vi "Pockels_FPGA.vi"(6 "Ethernet Port Opened ?":bool, 8 "error in (no error)":errorcluster, 9 "Laser(V)":dbl format="%#_13g", 10 "Pockels Mode_FPGA":T1(ring)=enum."Modulate", 11 "Imaging Protocol":T2=enum."Live Imaging") -> (0 "error out":errorcluster, 3 "Pockels Packet":string)   [LabVIEW 2020]
uses:
  Typedefs/Imaging Protocols enum.ctl
  Global Variables/General Globals.vi
panel:
  out "number":u32
  out "bin_in":bool[](array[boolean])
  out "bin_out_invert_14":bool[](array[boolean])
  out "Hex string 2":string
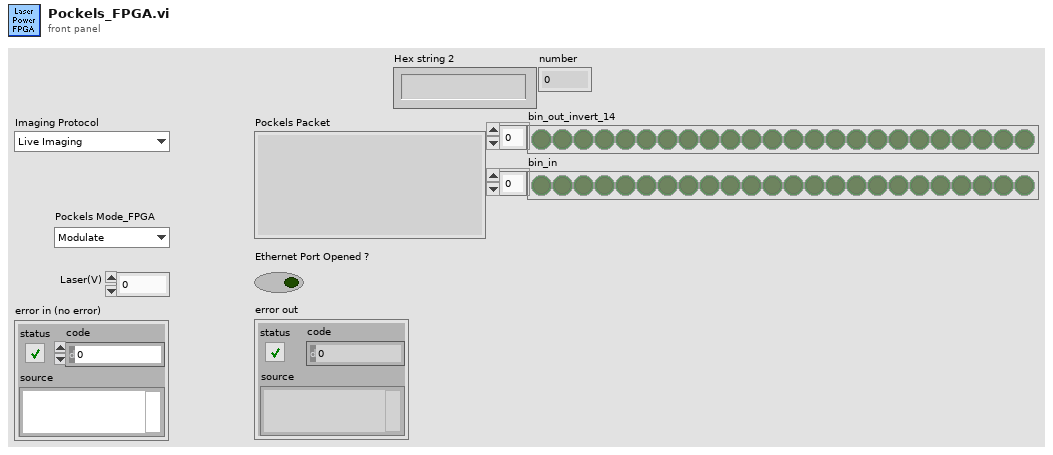
[diagram p1: front panel]
types:
  T1 = enum8{"Clear the register", "Always ON", "Modulate"}
  T2 = typedef "Imaging Protocols enum.ctl" = enum16{"AOL Z-Stack", "Motor Z Stack", "Functional Acquisition", "Single Plane Acquisition", "Volume Acquisition", "Live Imaging", "Live Plane Imaging", "Live Volume Imaging"}
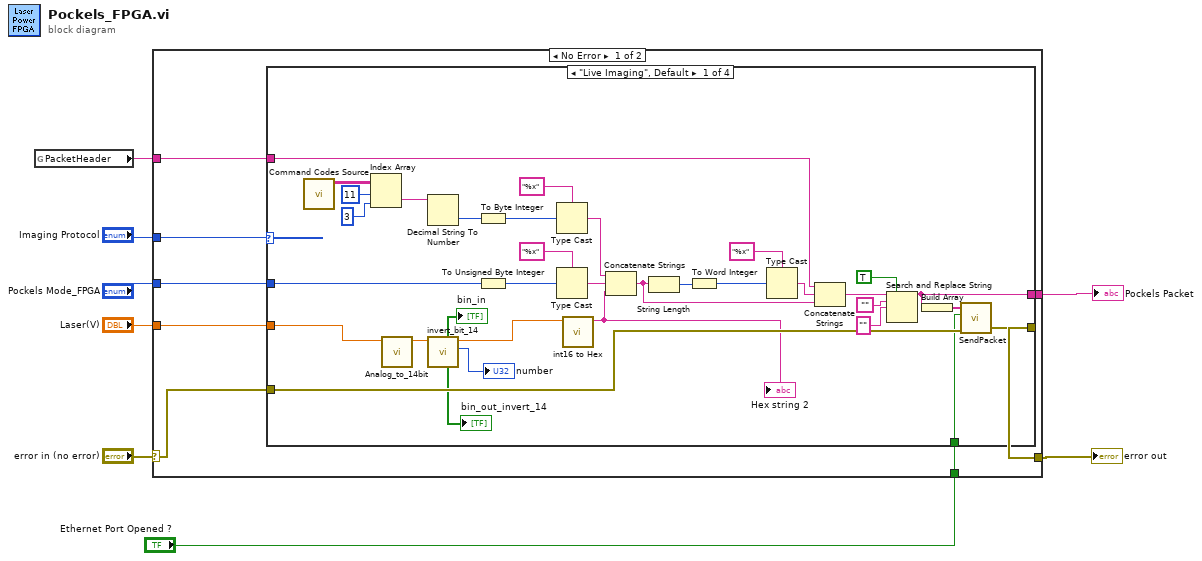
[diagram p0: block diagram]
diagram:
  n1 = global read "General Globals.vi" "PacketHeader"() -> (w3:string)
  n2 = case shown="No Error" "error in (no error)" {
    selector: "error in (no error)" -> [w10 w54]
    tunnel: "Imaging Protocol" -> [w16 _]
    tunnel: [w11 w54] -> w6
    tunnel: "Laser(V)" -> [w15 _]
    tunnel: "Pockels Mode_FPGA" -> [w14 _]
    tunnel: w3 -> [w13 _]
    tunnel: [w12 _] -> w2
    tunnel: "Ethernet Port Opened ?" -> [w9 _]
    frame No Error {
      n3 = case shown="\"Live Imaging\", Default" w16 {
        tunnel: w15 -> [w23 _ _ _]
        tunnel: w14 -> [w30 _ _ _]
        tunnel: w13 -> [w29 _ _ _]
        tunnel: [w27 _ _ _] -> w12
        tunnel: [w26 w51 w52 w53] -> w11
        tunnel: w10 -> [w25 w51 w52 w53]
        tunnel: w9 -> [w17 _ _ _]
        frame "Live Imaging", Default {
          n4 = call "Command Codes Source.vi"() -> ("Commands for FPGA"=w39:string[][])  [unwired: 11 in]
          n5 = Index Array(array=w39, index (row)=11 ("disabled index (row)"), index (col)=3 ("disabled index (col)")) -> (element=w42:string)
          n6 = call "Analog_to_14bit.vi"("Pockels (0-2V)"=w23) -> ("Pockels Level(14 bit)"=w22:dbl)  [unwired: 10 in]
          n7 = Decimal String To Number(string=w42) -> (number=w40:i32)  [unwired: 2 in, 1 out]
          n8 = call "invert_bit_14.vi"("Pockels Level(14 bit)"=w22) -> ("number"=→"number":u32, "to hex convert"=w21:dbl, "bin_out_invert_14"=→"bin_out_invert_14":bool[], "bin_in"=→"bin_in":bool[])  [unwired: 7 in]
          n9 = To Byte Integer(number=w40) -> (8bit integer=w41:i8)
          n10 = To Unsigned Byte Integer(number=w30) -> (unsigned 8bit integer=w48:u8)
          n11 = Type Cast(type="%x", x=w41) -> (*(type *) &x=w43:string)
          n12 = Type Cast(type="%x", x=w48) -> (*(type *) &x=w49:string)
          n13 = call "int16 to Hex.vi"("number"=w21) -> ("Hex string"=w24:string)  [unwired: 10 in]
          "Hex string 2" <- w24
          n14 = Concatenate Strings(w43, w49, w24) -> (w50:string)
          n15 = String Length(string=w50) -> (length=w44:i32)
          n16 = To Word Integer(number=w44) -> (16bit integer=w45:i16)
          n17 = Type Cast(type="%x", x=w45) -> (*(type *) &x=w46:string)
          n18 = Concatenate Strings(w29, w46, w50) -> (w47:string)
          n19 = Search and Replace String(replace all?=TRUE ("replace all? (F)"), input string=w47, search string="", replace string="" ("replace string (\"\")")) -> (result string=w27:string)  [unwired: 4 in, 3 out]
          n20 = Build Array(w27) -> (w28:string[])
          n21 = call "SendPacket.vi"("error in"=w25, "Ethernet Port Opened ?"=w17, "Packet Array"=w28) -> ("error out"=w26:errorcluster)  [unwired: 7 in, 1 out]
        }
        frame "AOL Z-Stack" {
        }
        frame "Functional Acquisition" {
        }
        frame "Motor Z Stack" {
        }
      }
    }
    frame Error {
    }
  }
  "error out" <- w6
  "Pockels Packet" <- w2
